vi "AllThingsImage.vi"   [LabVIEW 2024]
uses:
  <userlib>/ImageProcessing/FilterRedPlane.vi
  <userlib>/ImageProcessing/FilterGreenPlane.vi
  <userlib>/ImageProcessing/FilterBluePlane.vi
  <userlib>/ImageProcessing/InitCamera_NTSC.vi
  <userlib>/ImageProcessing/InitCamera_PAL.vi
  <userlib>/ImageProcessing/SaveMovieFile.vi
  <userlib>/ImageProcessing/IdentifyBlob_Square_Cluster.vi
  <userlib>/ImageProcessing/IdentifyBlob_Circle_Cluster.vi
  <userlib>/ImageProcessing/IdentifyBlob_Circle_Image.vi
  <userlib>/ImageProcessing/IdentifyBlob_Square_Image.vi
types:
  T1 = typedef "QT_Image.ctl" = cluster{"Width":i32, "Height":i32, "Depth":i32, "data":u8[], "Compressed data":u8[], "Color table":u32[], "Duration":i32, "Options":i32, "Timestamp":i32, "ID":i32, "Reserved":i32, "Dialogs":u32}
  T2 = typedef "QT_Ref.ctl" = refnum<k1>
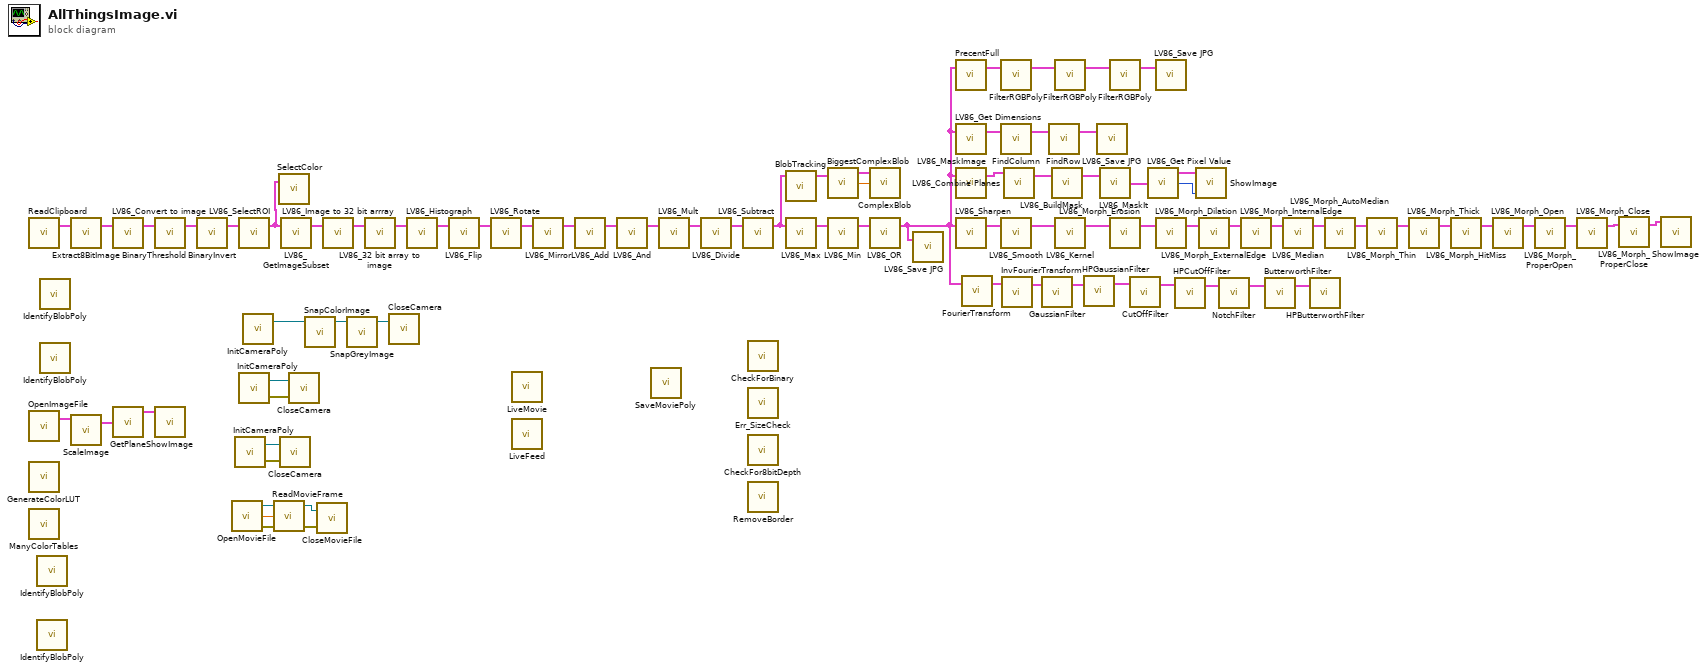
[diagram p0: block diagram]
diagram:
  n1 = call <userlib>:"ReadClipboard.vi"() -> ("Image Out"=w73:T1)  [unwired: 3 out]
  n2 = call <userlib>:"OpenImageFile.vi"() -> ("Image Out"=w76:T1)  [unwired: 1 in, 2 out]
  n3 = call <userlib>:"GenerateColorLUT.vi"() -> ()  [unwired: 5 out]
  n4 = call <userlib>:"ManyColorTables.vi"() -> ()  [unwired: 1 in, 3 out]
  n5 = call-poly <userlib>:"IdentifyBlobPoly.vi"() -> ()  [unwired: 4 in, 1 out]
  n6 = call-poly <userlib>:"IdentifyBlobPoly.vi"() -> ()  [unwired: 4 in, 1 out]
  n7 = call-poly <userlib>:"IdentifyBlobPoly.vi"() -> ()  [unwired: 4 in, 1 out]
  n8 = call-poly <userlib>:"IdentifyBlobPoly.vi"() -> ()  [unwired: 4 in, 1 out]
  n9 = call <userlib>:"Extract8BitImage.vi"("Image in"=w73) -> ("Image out"=w72:T1)  [unwired: 1 in, 1 out]
  n10 = call <userlib>:"ScaleImage.vi"("Image in"=w76) -> ("Image Out"=w75:T1)  [unwired: 4 in]
  n11 = call <userlib>:"LV86_Convert to image.vi"("Image In"=w72) -> ("Image Out"=w71:T1)  [unwired: 2 in]
  n12 = call <userlib>:"GetPlane.vi"("Image In"=w75) -> ("Red Plane Out"=w74:T1)  [unwired: 2 out]
  n13 = call <userlib>:"BinaryThreshold.vi"("Image In"=w71) -> ("Image Out"=w70:T1)  [unwired: 1 in, 1 out]
  n14 = call <userlib>:"ShowImage.vi"("Image"=w74) -> ()  [unwired: 2 in, 2 out]
  n15 = call <userlib>:"BinaryInvert.vi"("Image In"=w70) -> ("Image Out"=w69:T1)  [unwired: 2 out]
  n16 = call <userlib>:"OpenMovieFile.vi"() -> ("error out"=w21:errorcluster, "# frames"=w20:dbl, "QT Ref Out"=w19:T2)  [unwired: 1 in]
  n17 = call-poly <userlib>:"InitCameraPoly.vi"() -> ("error out"=w26:errorcluster, "QT Ref Out"=w25:T2)  [unwired: 2 in]
  n18 = call <userlib>:"LV86_SelectROI.vi"("Image"=w69) -> ("Image"=w10:T1)  [unwired: 2 out]
  n19 = call-poly <userlib>:"InitCameraPoly.vi"() -> ("error out"=w24:errorcluster, "QT Ref Out"=w23:T2)  [unwired: 2 in]
  n20 = call-poly <userlib>:"InitCameraPoly.vi"() -> ("QT Ref Out"=w27:T2)  [unwired: 2 in, 1 out]
  n21 = call <userlib>:"ReadMovieFrame.vi"("error in"=w21, "Frame Number"=w20, "QT Ref In"=w19) -> ("error out"=w18:errorcluster, "QT Ref Out"=w17:T2)  [unwired: 1 out]
  n22 = call <userlib>:"SelectColor.vi"("Image"=w10) -> ()  [unwired: 1 in, 2 out]
  n23 = call <userlib>:"CloseCamera.vi"("error in (no error)"=w26, "QT Ref In"=w25) -> ()  [unwired: 2 out]
  n24 = call <userlib>:"LV86_GetImageSubset.vi"("Image In"=w10) -> ("Image out"=w67:T1)  [unwired: 1 in, 1 out]
  n25 = call <userlib>:"CloseCamera.vi"("error in (no error)"=w24, "QT Ref In"=w23) -> ()  [unwired: 2 out]
  n26 = call <userlib>:"SnapColorImage.vi"("QT Ref In"=w27) -> ("QT Ref Out"=w55:T2)  [unwired: 1 in, 3 out]
  n27 = call <userlib>:"CloseMovieFile.vi"("error out"=w18, "QT Ref Out"=w17) -> ()  [unwired: 2 in]
  n28 = call <userlib>:"LV86_Image to 32 bit arrray.vi"("Image In"=w67) -> ("Image out"=w68:T1)  [unwired: 1 in, 1 out]
  n29 = call <userlib>:"SnapGreyImage.vi"("QT Ref In"=w55) -> ("QT Ref Out"=w54:T2)  [unwired: 1 in, 3 out]
  n30 = call <userlib>:"LV86_32 bit array to image.vi"("Image In"=w68) -> ("Image Out"=w62:T1)  [unwired: 2 in]
  n31 = call <userlib>:"CloseCamera.vi"("QT Ref In"=w54) -> ()  [unwired: 1 in, 2 out]
  n32 = call <userlib>:"LV86_Histograph.vi"("Image"=w62) -> ("Image Out"=w66:T1)  [unwired: 2 out]
  n33 = call <userlib>:"LV86_Flip.vi"("Image"=w66) -> ("Image"=w65:T1)  [unwired: 1 in, 1 out]
  n34 = call <userlib>:"LV86_Rotate.vi"("Image In"=w65) -> ("Image Out"=w64:T1)  [unwired: 1 in, 1 out]
  n35 = call <userlib>:"LiveMovie.vi"() -> ()  [unwired: 12 in]
  n36 = call <userlib>:"LiveFeed.vi"() -> ()  [unwired: 12 in]
  n37 = call <userlib>:"LV86_Mirror.vi"("Image"=w64) -> ("Image"=w63:T1)  [unwired: 2 out]
  n38 = call <userlib>:"LV86_Add.vi"("Image"=w63) -> ("Image Out"=w58:T1)  [unwired: 2 in]
  n39 = call <userlib>:"LV86_And.vi"("Image"=w58) -> ("Image Out"=w59:T1)  [unwired: 2 in]
  n40 = call-poly <userlib>:"SaveMoviePoly.vi"() -> ()  [unwired: 12 in]
  n41 = call <userlib>:"LV86_Mult.vi"("Image"=w59) -> ("Image Out"=w60:T1)  [unwired: 2 in]
  n42 = call <userlib>:"LV86_Divide.vi"("Image"=w60) -> ("Image Out"=w61:T1)  [unwired: 2 in]
  n43 = call <userlib>:"LV86_Subtract.vi"("Image"=w61) -> ("Image Out"=w16:T1)  [unwired: 2 in]
  n44 = call <userlib>:"CheckForBinary.vi"() -> ()  [unwired: 3 in, 1 out]
  n45 = call <userlib>:"Err_SizeCheck.vi"() -> ()  [unwired: 2 in, 2 out]
  n46 = call <userlib>:"CheckFor8bitDepth.vi"() -> ()  [unwired: 1 in, 3 out]
  n47 = call <userlib>:"RemoveBorder.vi"() -> ()  [unwired: 2 in, 1 out]
  n48 = call <userlib>:"BlobTracking.vi"("Image in"=w16) -> ("Image out"=w15:T1)  [unwired: 3 in, 3 out]
  n49 = call <userlib>:"LV86_Max.vi"("Image"=w16) -> ("Image Out"=w56:T1)  [unwired: 2 in]
  n50 = call <userlib>:"BiggestComplexBlob.vi"("Image in"=w15) -> ("Area"=w14:dbl, "Image out"=w13:T1)  [unwired: 1 in, 1 out]
  n51 = call <userlib>:"LV86_Min.vi"("Image"=w56) -> ("Image Out"=w57:T1)  [unwired: 2 in]
  n52 = call <userlib>:"ComplexBlob.vi"("Connectivity"=w14, "Image in"=w13) -> ()  [unwired: 1 in, 3 out]
  n53 = call <userlib>:"LV86_OR.vi"("Image"=w57) -> ("Image Out"=w9:T1)  [unwired: 2 in]
  n54 = call <userlib>:"LV86_Save JPG.vi"("Image"=w9) -> ()  [unwired: 1 in, 2 out]
  n55 = call <userlib>:"PrecentFull.vi"("Image In"=w9) -> ("Image Out"=w31:T1)  [unwired: 1 in, 1 out]
  n56 = call <userlib>:"LV86_Get Dimensions.vi"("Image In"=w9) -> ("Image Out"=w30:T1)  [unwired: 1 in, 1 out]
  n57 = call <userlib>:"LV86_MaskImage.vi"("Image"=w9) -> ("Image Out"=w53:T1)  [unwired: 1 in, 1 out]
  n58 = call <userlib>:"LV86_Sharpen.vi"("Image in"=w9) -> ("Image out"=w47:T1)  [unwired: 2 in]
  n59 = call <userlib>:"FourierTransform.vi"("Image In"=w9) -> ("Image Out"=w8:T1)  [unwired: 1 in, 1 out]
  n60 = call-poly <userlib>:"FilterRGBPoly.vi"("Image in"=w31) -> ("Image out"=w29:T1)  [unwired: 1 in, 1 out]
  n61 = call <userlib>:"FindColumn.vi"("Image In"=w30) -> ("Image Out"=w12:T1)  [unwired: 1 in, 1 out]
  n62 = call <userlib>:"LV86_Smooth.vi"("Image in"=w47) -> ("Image out"=w46:T1)  [unwired: 2 in]
  n63 = call <userlib>:"InvFourierTransform.vi"("Image In"=w8) -> ("Image Out"=w7:T1)  [unwired: 2 in]
  n64 = call <userlib>:"LV86_Combine Planes.vi"("Red"=w53) -> ("Image 2"=w52:T1)  [unwired: 2 in, 1 out]
  n65 = call <userlib>:"GaussianFilter.vi"("Image In"=w7) -> ("Image Out"=w6:T1)  [unwired: 1 in, 1 out]
  n66 = call <userlib>:"FindRow.vi"("Image In"=w12) -> ("Image Out"=w11:T1)  [unwired: 1 in, 1 out]
  n67 = call <userlib>:"LV86_BuildMask.vi"("Image"=w52) -> ("Image"=w51:T1)  [unwired: 1 in, 1 out]
  n68 = call-poly <userlib>:"FilterRGBPoly.vi"("Image in"=w29) -> ("Image out"=w28:T1)  [unwired: 1 in, 1 out]
  n69 = call <userlib>:"LV86_Kernel.vi"("Image in"=w46) -> ("Image out"=w45:T1)  [unwired: 2 in]
  n70 = call <userlib>:"HPGaussianFilter.vi"("Image In"=w6) -> ("Image Out"=w5:T1)  [unwired: 1 in, 1 out]
  n71 = call <userlib>:"LV86_Save JPG.vi"("Image"=w11) -> ()  [unwired: 1 in, 2 out]
  n72 = call <userlib>:"LV86_MaskIt.vi"("Image In"=w51) -> ("Image Out"=w50:T1)  [unwired: 1 in]
  n73 = call-poly <userlib>:"FilterRGBPoly.vi"("Image in"=w28) -> ("Image out"=w22:T1)  [unwired: 1 in, 1 out]
  n74 = call <userlib>:"LV86_Morph_Erosion.vi"("Image in"=w45) -> ("Image out"=w44:T1)  [unwired: 2 in]
  n75 = call <userlib>:"CutOffFilter.vi"("Image In"=w5) -> ("Image Out"=w4:T1)  [unwired: 1 in, 1 out]
  n76 = call <userlib>:"LV86_Get Pixel Value.vi"("Image In"=w50) -> ("I"=w49:u32, "Image Out"=w48:T1)  [unwired: 1 in, 2 out]
  n77 = call <userlib>:"LV86_Save JPG.vi"("Image"=w22) -> ()  [unwired: 1 in, 2 out]
  n78 = call <userlib>:"LV86_Morph_Dilation.vi"("Image in"=w44) -> ("Image out"=w43:T1)  [unwired: 2 in]
  n79 = call <userlib>:"HPCutOffFilter.vi"("Image In"=w4) -> ("Image Out"=w3:T1)  [unwired: 1 in, 1 out]
  n80 = call <userlib>:"ShowImage.vi"("Color Table"=w49, "Image"=w48) -> ()  [unwired: 1 in, 2 out]
  n81 = call <userlib>:"LV86_Morph_ExternalEdge.vi"("Image in"=w43) -> ("Image out"=w42:T1)  [unwired: 2 in]
  n82 = call <userlib>:"NotchFilter.vi"("Image In"=w3) -> ("Image Out"=w2:T1)  [unwired: 1 in, 1 out]
  n83 = call <userlib>:"LV86_Morph_InternalEdge.vi"("Image in"=w42) -> ("Image out"=w37:T1)  [unwired: 2 in]
  n84 = call <userlib>:"ButterworthFilter.vi"("Image In"=w2) -> ("Image Out"=w1:T1)  [unwired: 2 in, 1 out]
  n85 = call <userlib>:"LV86_Median.vi"("Image in"=w37) -> ("Image out"=w41:T1)  [unwired: 2 in]
  n86 = call <userlib>:"HPButterworthFilter.vi"("Image In"=w1) -> ()  [unwired: 2 in, 2 out]
  n87 = call <userlib>:"LV86_Morph_AutoMedian.vi"("Image in"=w41) -> ("Image out"=w40:T1)  [unwired: 2 in]
  n88 = call <userlib>:"LV86_Morph_Thin.vi"("Image in"=w40) -> ("Image out"=w39:T1)  [unwired: 2 in]
  n89 = call <userlib>:"LV86_Morph_Thick.vi"("Image in"=w39) -> ("Image out"=w38:T1)  [unwired: 2 in]
  n90 = call <userlib>:"LV86_Morph_HitMiss.vi"("Image in"=w38) -> ("Image out"=w36:T1)  [unwired: 2 in]
  n91 = call <userlib>:"LV86_Morph_Open.vi"("Image in"=w36) -> ("Image out"=w35:T1)  [unwired: 2 in]
  n92 = call <userlib>:"LV86_Morph_ProperOpen.vi"("Image in"=w35) -> ("Image out"=w34:T1)  [unwired: 2 in]
  n93 = call <userlib>:"LV86_Morph_Close.vi"("Image in"=w34) -> ("Image out"=w33:T1)  [unwired: 2 in]
  n94 = call <userlib>:"LV86_Morph_ProperClose.vi"("Image in"=w33) -> ("Image out"=w32:T1)  [unwired: 2 in]
  n95 = call <userlib>:"ShowImage.vi"("Image"=w32) -> ()  [unwired: 2 in, 2 out]
